vi "example 11 - tabs.vi"() -> ()   [LabVIEW 2020]
uses:
  ui-testing.lvlib
panel:
  out "Selected tab":string
  in  "Tab Control":enum32{"Page 1", "Page 2"}(tab)
  in  "tab button 1":bool
  in  "tab button 2":bool
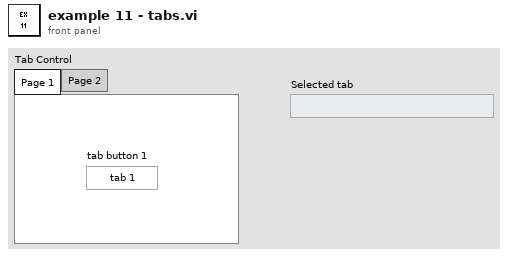
[diagram p1: front panel]
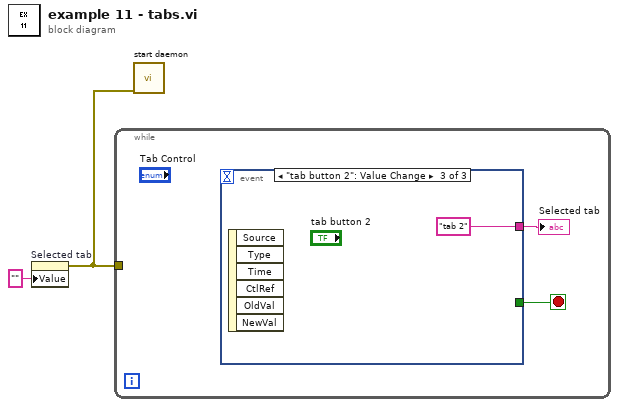
[diagram p0: block diagram]
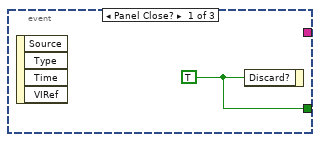
[diagram p2: hidden frame]
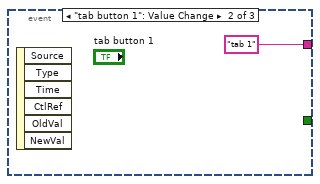
[diagram p3: hidden frame]
diagram:
  n1 = property on="Selected tab" class="Str"("Value"="" ("Selected tab")) -> (error out=w1:errorcluster)  [unwired: 2 in, 1 out]
  n2 = while {
    tunnel: w1 -> [_]
    stop <- w4 stop-if-true
    n3 = event shown="[2] \"tab button 2\": Value Change" {
      selector: _ -> [_ _ _]
      dyn-events: _ -> [_ _ _]
      timeout: _ -> [_ _ _]
      tunnel: [w5 _ _] -> w4
      tunnel: [_ "tab 1" "tab 2"] -> w3
      event Panel Close? {
        w5 = TRUE
        n4 = event-data() -> ()  [unwired: 1 in, 4 out]
        n5 = event-data("Discard?"=w5) -> ()  [unwired: 1 in, 1 out]
      }
      event "tab button 1": Value Change {
        n6 = event-data() -> ()  [unwired: 1 in, 6 out]
      }
      event "tab button 2": Value Change {
        n7 = event-data() -> ()  [unwired: 1 in, 6 out]
      }
    }
    "Selected tab" <- w3
  }
  n8 = call "start daemon.vi"("error in (no error)"=w1) -> ()  [unwired: 10 in, 1 out]
